vi "Configure Channels.vi"(8 "error in":errorcluster, 11 "DAQmx Thermocouple Continuous Read Strategy in":refnum<class "DAQmx Thermocouple Continuous Read Strategy.lvclass">) -> (0 "error out":errorcluster, 3 "DAQmx Thermocouple Continuous Read Strategy out":refnum<class "DAQmx Thermocouple Continuous Read Strategy.lvclass">)   [LabVIEW 2024, in "DAQmx Thermocouple Continuous Read Strategy.lvclass"]
uses:
  DAQmx Thermocouple Continuous Read Strategy.lvclass
  D:/git/HAL/HAL-Devices/Source/DAQmx Base Configure Strategy/DAQmx Base Configure Strategy.lvclass
  DAQmx Base Configure Strategy/DAQmx Base Configure Strategy.lvclass/DAQmx Base Configure Strategy.ctl
  <vilib>/JDP Science/JSONtext/LVClass Serializer/JSONtext LVClass Serializer.lvclass
  Source/Interfaces/IConfiguration/IConfiguration.lvclass
  DAQmx Base Configure Strategy/DAQmx Base Configure Strategy.lvclass
  3bccc76a-65ad-40c9-85ac-8ed8ddce32d9.vi
  <vilib>/DAQmx/create/channels.llb/DAQmx Create Channel (AI-Temperature-Thermocouple).vi
panel:
  out "units":i32(ring)=10143 items=["Deg C"=10143, "Deg F"=10144, "Kelvins"=10325, "Deg R"=10145, "From Custom Scale"=10065]
  out "cjc source":i32(ring)=10116 items=["Built-In"=10200, "Constant Value"=10116, "Channel"=10113]
  out "thermocouple type":i32(ring)=10072 items=["J"=10072, "K"=10073, "N"=10077, "R"=10082, "S"=10085, "T"=10086, "B"=10047, "E"=10055]
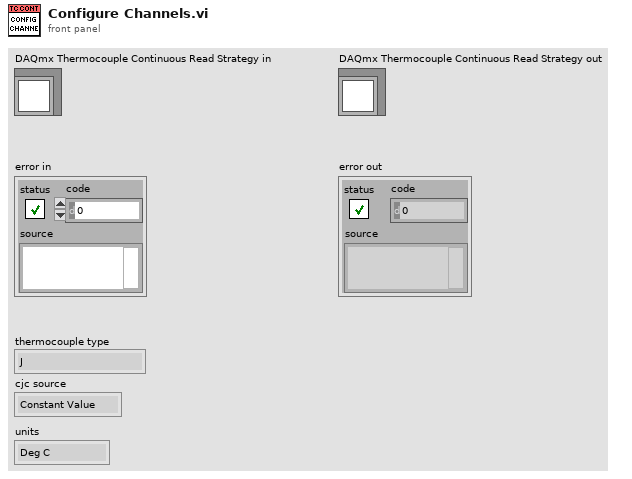
[diagram p1: front panel]
types:
  T1 = cluster{"Name":string, "Enabled":bool, "Minimum Value":dbl, "Maximum Value":dbl, "Thermocouple Type":string, "Units":string, "CJC Channel":string, "CJC Source":string, "CJC Value":dbl}[]
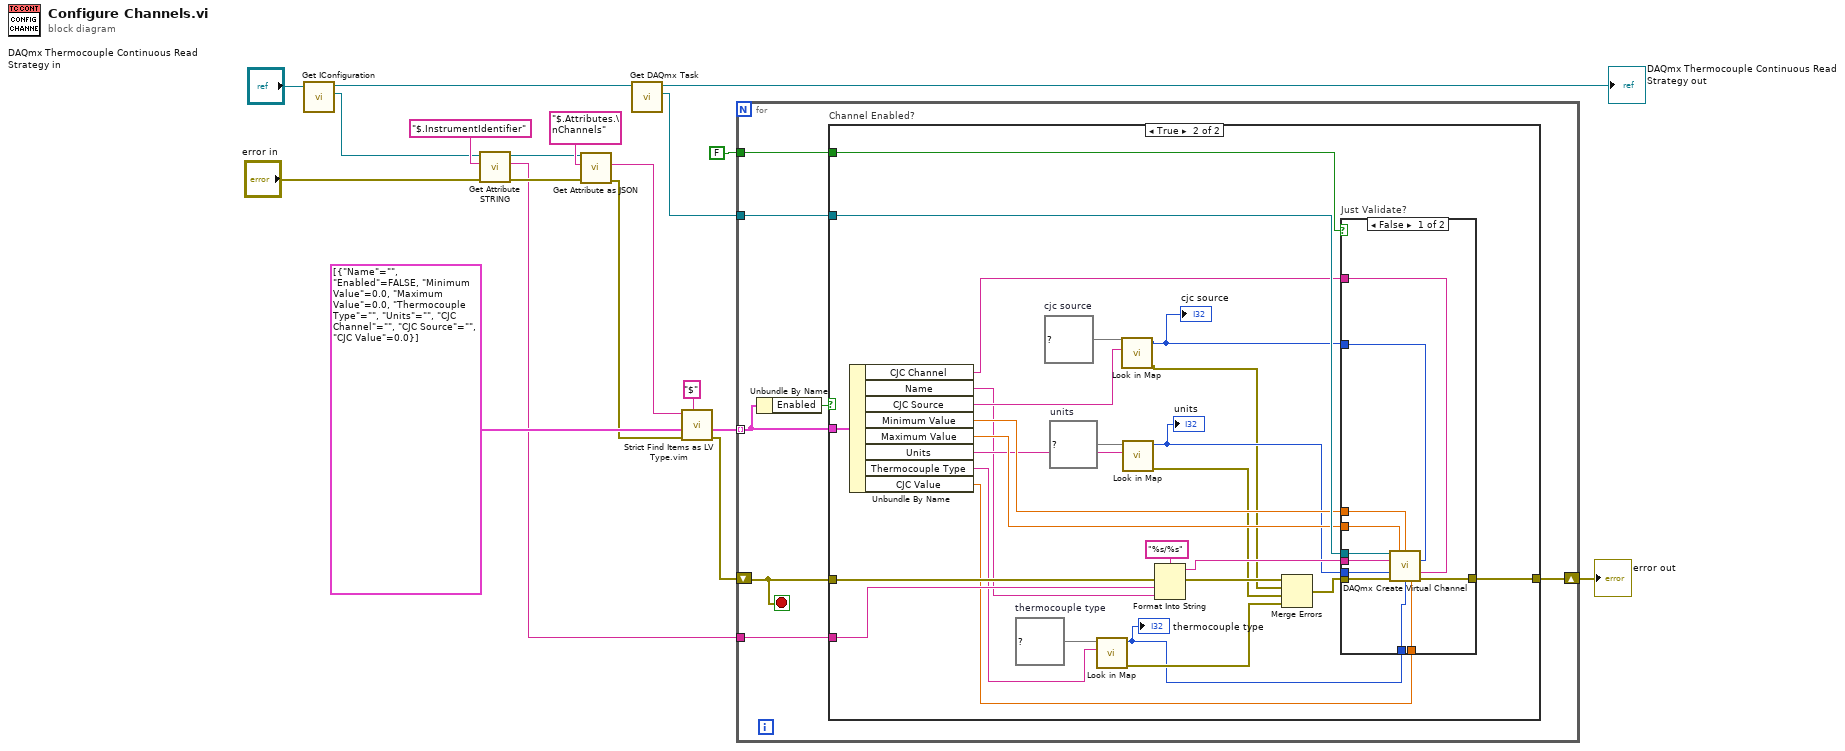
[diagram p0: block diagram]
diagram:
  n1 = call-dynamic "Get IConfiguration.vi"("DAQmx Base Configure Strategy in"="DAQmx Thermocouple Continuous Read Strategy in") -> ("IConfiguration"=w7:refnum<class "IConfiguration.lvclass">, "DAQmx Base Configure Strategy out"=w8:refnum<class "DAQmx Thermocouple Continuous Read Strategy.lvclass">)  [unwired: 9 in]
  n2 = call-dynamic "Get Attribute STRING.vi"("error in"="error in", "Attribute"="$.InstrumentIdentifier", "IConfiguration in"=w7) -> ("error out"=w12:errorcluster, "Value"=w10:string, "IConfiguration out"=w13:refnum<class "IConfiguration.lvclass">)  [unwired: 6 in]
  n3 = call-dynamic "Get Attribute as JSON.vi"("error in"=w12, "Attribute"="$.Attributes.\nChannels", "IConfiguration in"=w13) -> ("error out"=w15:errorcluster, "<JSON>"=w18:string)  [unwired: 6 in, 1 out]
  n4 = call "Get DAQmx Task.vi"("DAQmx Base Configure Strategy in"=w8) -> ("DAQmx Task"=w6:refnum<k21>, "DAQmx Base Configure Strategy out"=→"DAQmx Thermocouple Continuous Read Strategy out":refnum<class "DAQmx Thermocouple Continuous Read Strategy.lvclass">)  [unwired: 9 in]
  n5 = call "Strict Find Items as LV Type.vim"("$Path or Item Name"="$", "error in"=w15, "Data Type and Default Value"=T1 [{"Name"="", "Enabled"=FALSE, "Minimum Value"=0.0, "Maximum Value"=0.0, "Thermocouple Type"="", "Units"="", "CJC Channel"="", "CJC Source"="", "CJC Value"=0.0}], "<JSON>"=w18) -> ("error out"=w14:errorcluster, "Data out"=w16:T1)  [unwired: 5 in, 1 out]
  n6 = for {
    tunnel: w16 -> [w23] mode=indexing
    shift-right: [w26] -> w3
    shift-left: w14 -> [w25]
    tunnel: w10 -> [w24]
    tunnel: FALSE -> [w20]
    tunnel: w6 -> [w22]
    stop <- w25 stop-if-true
    n7 = Unbundle By Name(w23) -> ("Enabled"=w21:bool)
    n8 = case "Channel Enabled?" shown="True" w21 {
      tunnel: [w27 w29] -> w26
      tunnel: w25 -> [w27 w51]
      tunnel: w24 -> [_ w50]
      tunnel: w23 -> [_ w54]
      tunnel: w22 -> [_ w53]
      tunnel: w20 -> [_ w28]
      frame False {
      }
      frame True {
        w35 = map{string, i32} {"B"=10047, "E"=10055, "J"=10072, "K"=10073, "N"=10077, "R"=10082, "S"=10085, "T"=10086}  # thermocouple type
        w36 = map{string, i32} {"Built-In"=10200, "Channel"=10113, "Constant Value"=10116}  # cjc source
        w44 = map{string, i32} {"Deg C"=10143, "Deg F"=10144, "Deg R"=10145, "From Custom Scale"=10065, "Kelvins"=10325}  # units
        n9 = Unbundle By Name(w54) -> ("CJC Channel"=w31:string, "Name"=w30:string, "CJC Source"=w38:string, "Minimum Value"=w46:dbl, "Maximum Value"=w45:dbl, "Units"=w42:string, "Thermocouple Type"=w40:string, "CJC Value"=w32:dbl)
        n10 = call "Look in Map.vi"("Key"=w40, "Map"=w35) -> ("error out"=w39:errorcluster, "Value"=w33:i32)  [unwired: 8 in]
        "thermocouple type" <- w33
        n11 = call "Look in Map.vi"("Key"=w38, "Map"=w36) -> ("error out"=w37:errorcluster, "Value"=w34:i32)  [unwired: 8 in]
        "cjc source" <- w34
        n12 = call "Look in Map.vi"("Key"=w42, "Map"=w44) -> ("error out"=w41:errorcluster, "Value"=w43:i32)  [unwired: 8 in]
        "units" <- w43
        n13 = Format Into String(format string="%s/%s", error in=w51, w50, w30) -> (resulting string=w48:string, error out=w49:errorcluster)  [unwired: 1 in]
        n14 = Merge Errors(w49, w37, w41, w39) -> (w47:errorcluster)
        n15 = case "Just Validate?" shown="False" w28 {
          tunnel: w47 -> [w58 w66]
          tunnel: w48 -> [w63 _]
          tunnel: w53 -> [w65 _]
          tunnel: [w64 w66] -> w29
          tunnel: w34 -> [w60 _]
          tunnel: w46 -> [w62 _]
          tunnel: w45 -> [w61 _]
          tunnel: w43 -> [w59 _]
          tunnel: w33 -> [w56 _]
          tunnel: w32 -> [w57 _]
          tunnel: w31 -> [w55 _]
          frame False {
            n16 = call-poly <vilib>:"DAQmx Create Virtual Channel.vi"("task in"=w65, "maximum value"=w61, "minimum value"=w62, "physical channels"=w63, "cjc source"=w60, "units"=w59, "cjc channel"=w55, "error in"=w58, "thermocouple type"=w56, "cjc value"=w57) -> ("error out"=w64:errorcluster)  [unwired: 4 in, 1 out]
          }
          frame True {
          }
        }
      }
    }
  }
  "error out" <- w3
